vi "Preview Execution Type.vi"(8 "error in (no error)":errorcluster, 10 "Flattened Linked List":string, 11 "IPersist in":refnum<class "IPersist.lvclass">) -> (0 "error out":errorcluster, 1 "Found?":bool, 2 "Flattened Linked List out":string, 3 "IPersist out":refnum<class "IPersist.lvclass">, 5 "Execution Type":refnum<class "Executioner.lvclass">)   [LabVIEW 2019, in "Test Executive.lvlib" / "Executioner.lvclass"]
uses:
  <vilib>/gpm_packages/@cs/test-executive/Source/Test Executive/Executioner/Executioner.lvclass
  <vilib>/gpm_packages/@cs/persistence/source/IPersist/IPersist.lvclass
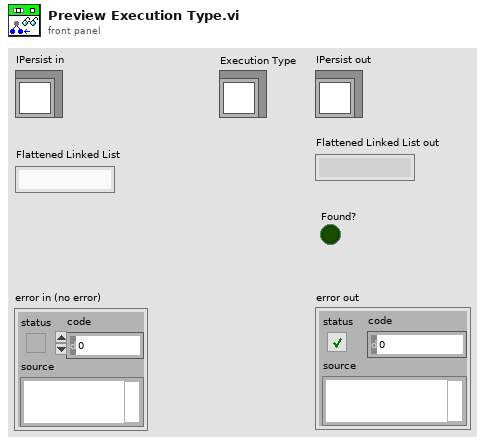
[diagram p1: front panel]
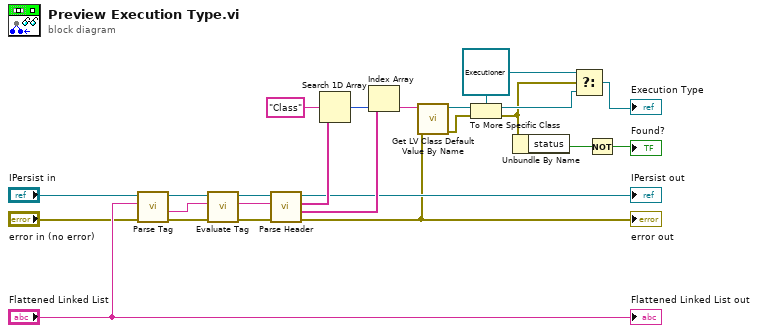
[diagram p0: block diagram]
diagram:
  w7 = refnum<class "Executioner.lvclass"> refnum ("Test Executive.lvlib:Executioner.lvclass")
  n1 = call-dynamic "Parse Tag.vi"("error in (no error)"="error in (no error)", "Flattened Linked List"="Flattened Linked List", "IPersist in"="IPersist in") -> ("error out"=w23:errorcluster, "Tag"=w12:string, "IPersist out"=w22:refnum<class "IPersist.lvclass">)  [unwired: 2 in, 4 out]
  n2 = call-dynamic "Evaluate Tag.vi"("error in (no error)"=w23, "Tag"=w12, "IPersist in"=w22) -> ("error out"=w4:errorcluster, "Header"=w20:string, "IPersist out"=w21:refnum<class "IPersist.lvclass">)  [unwired: 3 in, 3 out]
  "error out" <- w4
  n3 = call-dynamic "Parse Header.vi"("Header"=w20, "IPersist in"=w21) -> ("Value"=w17:string[], "Name"=w19:string[], "IPersist out"=→"IPersist out":refnum<class "IPersist.lvclass">)  [unwired: 7 in]
  n4 = Search 1D Array(1D array=w19, element="Class") -> (index of element=w16:i32)  [unwired: 1 in]
  n5 = Index Array(array=w17, index=w16) -> (element=w13:string)
  n6 = call <vilib>:"Get LV Class Default Value By Name.vi"("error in (no error)"=w4, "class name"=w13) -> ("error out"=w14:errorcluster, "object"=w15:refnum<class>)  [unwired: 8 in]
  n7 = To More Specific Class(target class=w7, reference=w15, error in=w14) -> (specific class reference=w6:refnum<class "Executioner.lvclass">, error out=w3:errorcluster)
  n8 = Unbundle By Name(w3) -> ("status"=w2:bool)
  n9 = Select(t=w7, s=w3, f=w6) -> (s? t:f=→"Execution Type":refnum<class "Executioner.lvclass">)
  n10 = Not(x=w2) -> (.not. x?=→"Found?":bool)
  "Flattened Linked List out" <- "Flattened Linked List"
